vi "Multidot SPC tracking.vi"() -> ()   [LabVIEW 2012]
panel:
  in  "Z interval (min)":dbl=10.0
  in  "Scan Interval (minutes)":dbl=2.0
  in  "Collection Time (hours)":dbl=3.0
  in  "File Path Control":path
  in  "Z Position 2":dbl
  in  "Y Parameters":T1={"Number of Y Steps"=200, "Max Y (V)"=2.0, "Min Y (V)"=-2.0}
  in  "X Parameters":T2={"Number of X Steps"=200, "Max X (V)"=2.0, "Min X (V)"=-2.0}
  in  "RS232 settings":cluster{"Portnumber":i32, "Baudrate":u16}={"Portnumber"=6, "Baudrate"=5} {"Portnumber" items=["COM1", "COM2", "COM3", "COM4", "COM5", "COM6", "COM7", "COM8", "COM9", "COM10", "COM11", "COM12", "COM13", "COM14", "COM15", "COM16", "COM17", "COM18", "COM19", "COM20", "COM21", "COM22", "COM23", "COM24", "COM25", "COM26", "COM27", "COM28", "COM29", "COM30"]; "Baudrate" items=["9600", "14400", "19200", "38400", "57600", "115200"]}
  in  "stop":bool
  in  "Array - Numeric":dbl[][](array[numeric])=[[0.0, 0.0], [0.0, 0.0], [0.0, 0.0], [0.0, 0.0], [0.0, 0.0], [0.0, 0.0]]
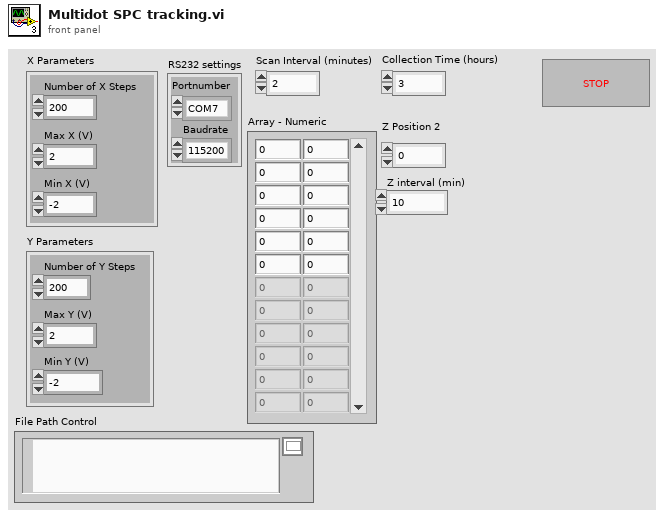
[diagram p1: front panel]
types:
  T1 = cluster{"Number of Y Steps":i32, "Max Y (V)":dbl, "Min Y (V)":dbl}
  T2 = cluster{"Number of X Steps":i32, "Max X (V)":dbl, "Min X (V)":dbl}
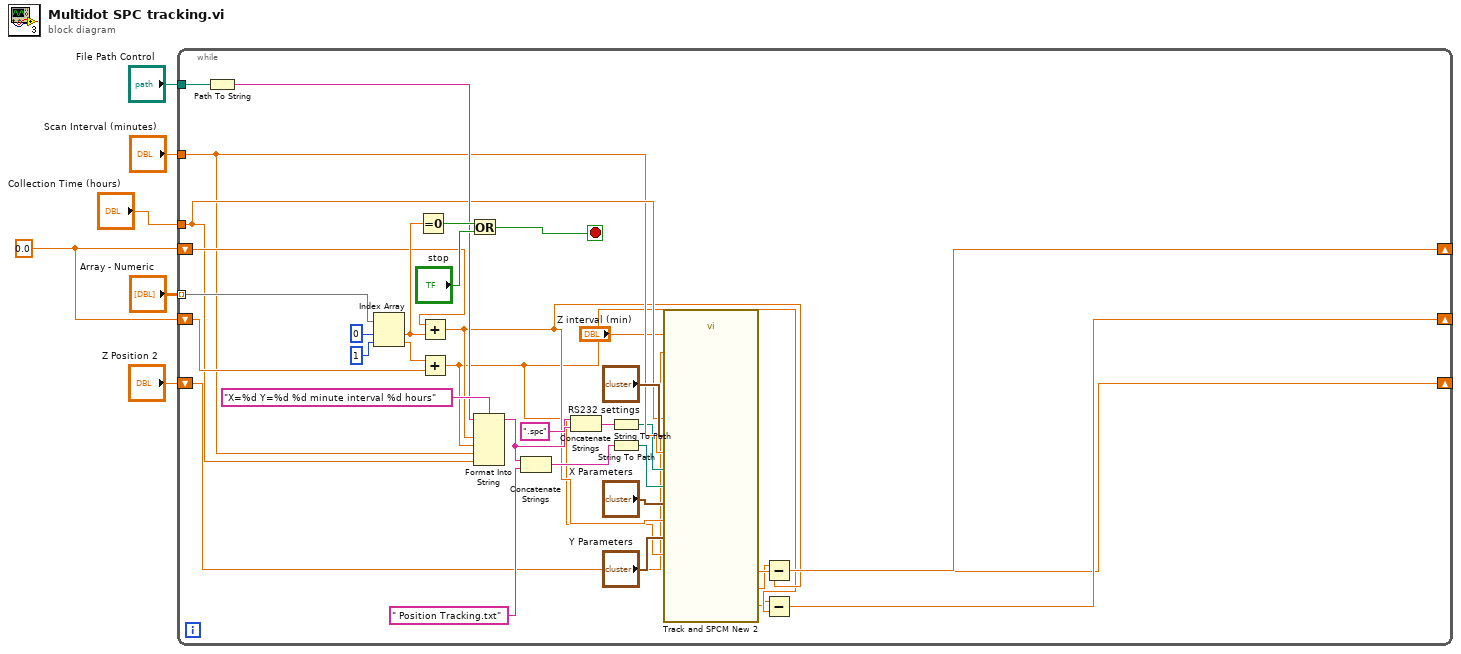
[diagram p0: block diagram]
diagram:
  w1 = 0.0 ("Result")
  n1 = while {
    tunnel: "Array - Numeric" -> [w40] mode=indexing
    shift-right: [w10] -> _
    shift-left: "Z Position 2" -> [w11]
    tunnel: "File Path Control" -> [w34]
    tunnel: "Collection Time (hours)" -> [w19]
    tunnel: "Scan Interval (minutes)" -> [w18]
    shift-right: [w24] -> _
    shift-left: w1 -> [w25]
    shift-right: [w23] -> _
    shift-left: w1 -> [w21]
    stop <- w36 stop-if-true
    n2 = Path To String(path=w34) -> (string=w27:string)
    n3 = Index Array(array=w40, index #1=0 ("index"), index #2=1 ("index")) -> (element #1=w26:dbl, element #2=w22:dbl)
    n4 = Equal To 0?(x=w26) -> (x = 0?=w35:bool)
    n5 = Add(x=w25, y=w26) -> (x+y=w13:dbl)
    n6 = Add(x=w22, y=w21) -> (x+y=w12:dbl)
    n7 = Or(x=w35, y="stop") -> (x .or. y?=w36:bool)
    n8 = Format Into String(format string="X=%d Y=%d %d minute interval %d hours", initial string=w27, w13, w12, w18, w19) -> (resulting string=w29:string)  [unwired: 1 in, 1 out]
    n9 = Concatenate Strings(w29, " Position Tracking.txt" ("string")) -> (w30:string)
    n10 = Concatenate Strings(w29, ".spc" ("string")) -> (w31:string)
    n11 = String To Path(string=w31) -> (path=w17:path)
    n12 = String To Path(string=w30) -> (path=w16:path)
    n13 = call "Track and SPCM New 2.vi"("X Parameters"="X Parameters", "X Pos"=w13, "Scan Interval (minutes)"=w18, "Y pos"=w12, "Y Parameters"="Y Parameters", "Z interval (min)"="Z interval (min)", "RS232 settings"="RS232 settings", "Z Pos"=w11, "SPCM File Path"=w17, "Collection Time (hours)"=w19, "Tracking Data File Path"=w16) -> ("X Position"=w8:dbl, "Y Position"=w9:dbl, "Z Position"=w10:dbl)  [unwired: 2 in]
    n14 = Subtract(x=w8, y=w13) -> (x-y=w24:dbl)
    n15 = Subtract(x=w9, y=w12) -> (x-y=w23:dbl)
  }
